vi "Car Race Message.vi"(7 "?":T1=enum."Game Over", 8 "error in":errorcluster) -> (0 "error IO":errorcluster, 2 "Message":string)   [LabVIEW 2013]
uses:
  Controls/Car race Msg.ctl
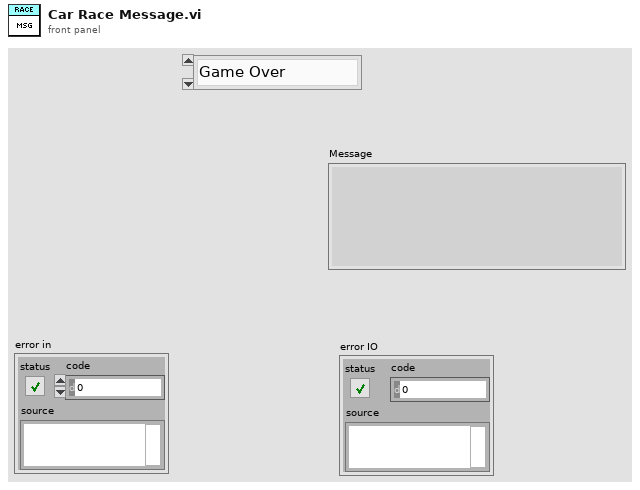
[diagram p1: front panel]
types:
  T1 = typedef "Car race Msg.ctl" = enum16{"Welcome Messsage", "User Inf.", "Start", "Log In Failed", "Game Over"}
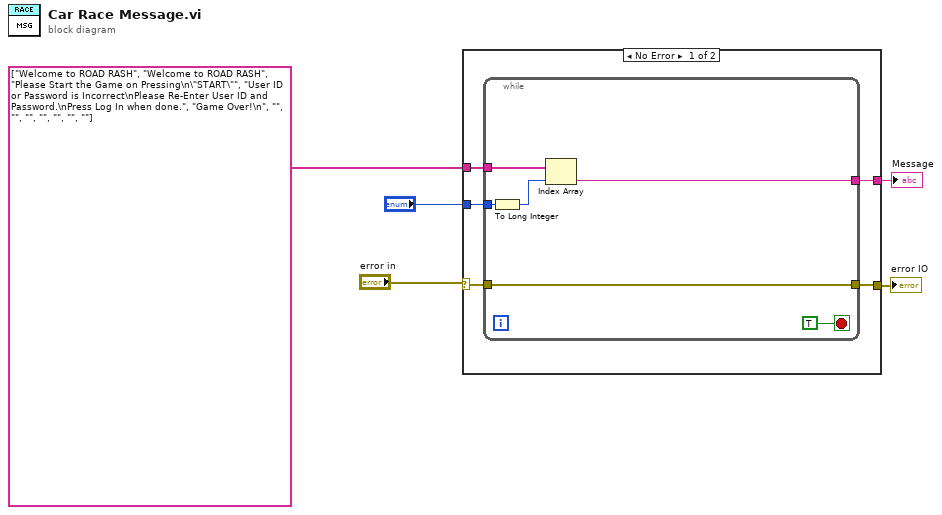
[diagram p0: block diagram]
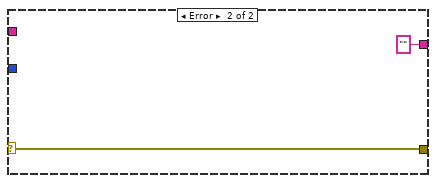
[diagram p2: hidden frame]
diagram:
  n1 = case shown="No Error" "error in" {
    selector: "error in" -> [w6 w18]
    tunnel: "?" -> [w10 _]
    tunnel: string[] ["Welcome to ROAD RASH", "Welcome to ROAD RASH", "Please Start the Game on Pressing\n\"START\"", "User ID or Password is Incorrect\nPlease Re-Enter User ID and Password.\nPress Log In when done.", "Game Over!\n", "", "", "", "", "", "", ""] -> [w9 _]
    tunnel: [w8 ""] -> w4
    tunnel: [w7 w18] -> w2
    frame No Error {
      n2 = while {
        tunnel: w10 -> [w15]
        tunnel: [w14] -> w8
        tunnel: w9 -> [w13]
        tunnel: [w12] -> w7
        tunnel: w6 -> [w12]
        stop <- TRUE stop-if-true
        n3 = To Long Integer(number=w15) -> (32bit integer=w11:i32)
        n4 = Index Array(array=w13, index=w11) -> (element=w14:string)
      }
    }
    frame Error {
    }
  }
  "Message" <- w4
  "error IO" <- w2
